vi "Color Sensor V3 Delta E.vi"(10 "CIE Lab 2":cluster{"L":dbl, "a":dbl, "b":dbl}, 11 "CIE Lab":cluster{"L":dbl, "a":dbl, "b":dbl}) -> (3 "CIE Delta E":dbl)   [LabVIEW 2019]
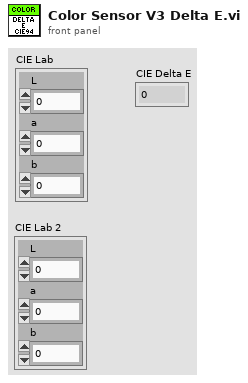
[diagram p1: front panel]
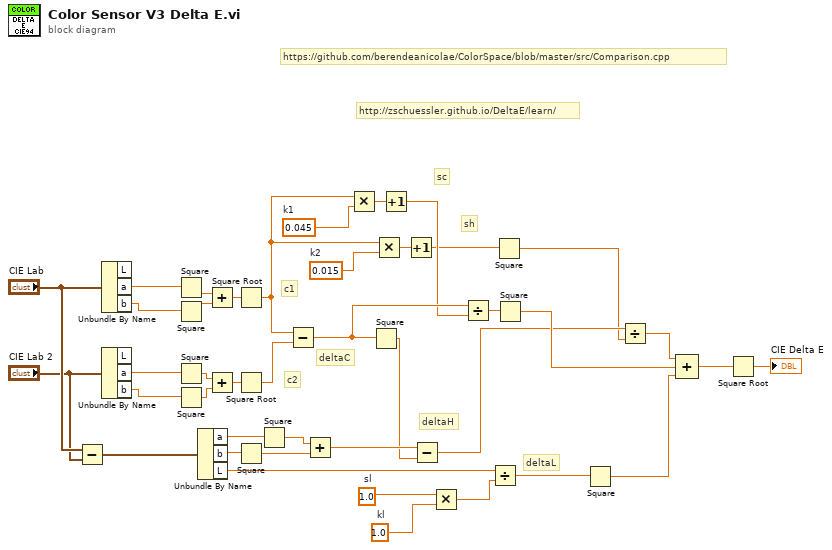
[diagram p0: block diagram]
diagram:
  w15 = 1.0  # kl
  w13 = 1.0  # sl
  w20 = 0.015  # k2
  w21 = 0.045  # k1
  # "https://github.com/berendeanicolae/ColorSpace/blob/master/src/Comparison.cpp"
  # "deltaL"
  # "deltaC"
  # "sh"
  # "sc"
  # "deltaH"
  # "c2"
  # "c1"
  # "http://zschuessler.github.io/DeltaE/learn/"
  n1 = Subtract(x="CIE Lab", y="CIE Lab 2") -> (x-y=w28:cluster{"L":dbl, "a":dbl, "b":dbl})
  n2 = Unbundle By Name("CIE Lab") -> ("a"=w39:dbl, "b"=w38:dbl)  [unwired: 1 out]
  n3 = Unbundle By Name("CIE Lab 2") -> ("a"=w37:dbl, "b"=w36:dbl)  [unwired: 1 out]
  n4 = Square(x=w39) -> (x^2=w34:dbl)
  n5 = Square(x=w38) -> (x^2=w35:dbl)
  n6 = Square(x=w37) -> (x^2=w31:dbl)
  n7 = Square(x=w36) -> (x^2=w30:dbl)
  n8 = Unbundle By Name(w28) -> ("a"=w27:dbl, "b"=w26:dbl, "L"=w17:dbl)
  n9 = Add(x=w34, y=w35) -> (x+y=w33:dbl)
  n10 = Add(x=w31, y=w30) -> (x+y=w32:dbl)
  n11 = Square Root(x=w33) -> (sqrt(x)=w16:dbl)
  n12 = Square Root(x=w32) -> (sqrt(x)=w29:dbl)
  n13 = Square(x=w26) -> (x^2=w22:dbl)
  n14 = Square(x=w27) -> (x^2=w23:dbl)
  n15 = Subtract(x=w16, y=w29) -> (x-y=w12:dbl)
  n16 = Add(x=w23, y=w22) -> (x+y=w25:dbl)
  n17 = Multiply(x=w16, y=w21) -> (x*y=w19:dbl)
  n18 = Square(x=w12) -> (x^2=w24:dbl)
  n19 = Multiply(x=w16, y=w20) -> (x*y=w18:dbl)
  n20 = Increment(x=w19) -> (x+1=w11:dbl)
  n21 = Increment(x=w18) -> (x+1=w6:dbl)
  n22 = Subtract(x=w25, y=w24) -> (x-y=w5:dbl)
  n23 = Multiply(x=w13, y=w15) -> (x*y=w14:dbl)
  n24 = Divide(x=w12, y=w11) -> (x/y=w10:dbl)
  n25 = Divide(x=w17, y=w14) -> (x/y=w9:dbl)
  n26 = Square(x=w6) -> (x^2=w4:dbl)
  n27 = Square(x=w10) -> (x^2=w7:dbl)
  n28 = Square(x=w9) -> (x^2=w8:dbl)
  n29 = Divide(x=w5, y=w4) -> (x/y=w3:dbl)
  n30 = Compound Arithmetic op=ADD(w3, w7, w8) -> (w2:dbl)
  n31 = Square Root(x=w2) -> (sqrt(x)=→"CIE Delta E":dbl)
